vi "Change Color Luminance.vi"(10 "New Grey Value (0-255)":u8, 11 "Color in":u32(colorbox)) -> (3 "Color out":u32(colorbox)=16777215)   [LabVIEW 2015, in "ColorSelector.lvclass"]
doc: "This VI will change the Luminance of the input color based off the input Grey Scale Value.\n\n0 Black\n0<x<=50 Dark variations of the Color\n50<x<=255 Light variations of the Color\n255 White\n<b> </b> <b> </b>\n©2017 Q Software Innovations, LLC (QSI)\nwritten by Quentin Alldredge\nproduced in LabVIEW 2015\n\nsupport@qsoftwareinnovations.com\nwww.qsoftwareinnovations.com\n\nAll rights reserved.\n\nRedistribution and use in source and binary forms, with or without modification, are permitted provided that the following conditions are met:\n\n * Redistributions of source code must retain the above copyright notice, this list of conditions and the following disclaimer.\n * Redistributions in binary form must reproduce the above copyright notice, this list of conditions and the following disclaimer in the documentation and/or other materials provided with the distribution.\n * Neither the name of Q Software Innovations, LLC. nor the names of its contributors may be used to endorse or promote products derived from this software without specific prior written permission.\n\nTHIS SOFTWARE IS PROVIDED BY THE COPYRIGHT HOLDERS AND CONTRIBUTORS \"AS IS\" AND ANY EXPRESS OR IMPLIED WARRANTIES, INCLUDING, BUT NOT LIMITED TO, THE IMPLIED WARRANTIES OF MERCHANTABILITY AND FITNESS FOR A PARTICULAR PURPOSE ARE DISCLAIMED. IN NO EVENT SHALL THE COPYRIGHT OWNER OR CONTRIBUTORS BE LIABLE FOR ANY DIRECT, INDIRECT, INCIDENTAL, SPECIAL, EXEMPLARY, OR CONSEQUENTIAL DAMAGES (INCLUDING, BUT NOT LIMITED TO, PROCUREMENT OF SUBSTITUTE GOODS OR SERVICES; LOSS OF USE, DATA, OR PROFITS; OR BUSINESS INTERRUPTION) HOWEVER CAUSED AND ON ANY THEORY OF LIABILITY, WHETHER IN CONTRACT, STRICT LIABILITY, OR TORT (INCLUDING NEGLIGENCE OR OTHERWISE) ARISING IN ANY WAY OUT OF THE USE OF THIS SOFTWARE, EVEN IF ADVISED OF THE POSSIBILITY OF SUCH DAMAGE."
uses:
  ColorSelector.lvclass
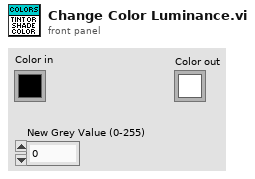
[diagram p1: front panel]
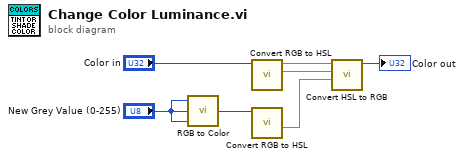
[diagram p0: block diagram]
diagram:
  n1 = call <vilib>:"RGB to Color.vi"("B"="New Grey Value (0-255)", "G"="New Grey Value (0-255)", "R"="New Grey Value (0-255)") -> ("Color"=w4:u32)
  n2 = call "Convert RGB to HSL.vi"("Color Box"="Color in") -> ("S (%)"=w1:dbl, "H (deg)"=w5:dbl)  [unwired: 8 in, 1 out]
  n3 = call "Convert RGB to HSL.vi"("Color Box"=w4) -> ("L (%)"=w2:dbl)  [unwired: 8 in, 2 out]
  n4 = call "Convert HSL to RGB.vi"("L (%)"=w2, "S (%)"=w1, "H (deg)"=w5) -> ("Color Box"=→"Color out":u32)  [unwired: 8 in]
